vi "Save Last Sync to File.vi"(8 "error in (no error)":errorcluster, 11 "Data Manager in":refnum<class "Data Manager.lvclass">) -> (0 "error out":errorcluster, 3 "Data Manager out":refnum<class "Data Manager.lvclass">)   [LabVIEW 2020, in "Data Manager.lvclass"]
uses:
  Data Manager.lvclass
  Data Manager.lvclass/Data Manager.ctl
  <vilib>/drjdpowell/SQLite Library/SQL Connection/Execute SQL (No results).vi
  <vilib>/drjdpowell/SQLite Library/SQLite.lvlib
  <vilib>/drjdpowell/SQLite Library/SQL Connection/Connection.lvclass
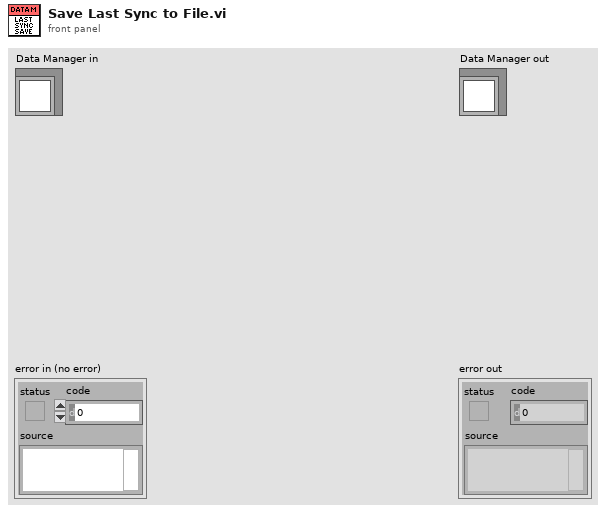
[diagram p1: front panel]
types:
  T1 = typedef "Data Manager.lvclass/Strava JSON for Club Activities--cluster.ctl" = cluster{"athlete":cluster{"firstname":string, "lastname":string}, "type":string, "distance":dbl, "moving_time":dbl, "elapsed_time":dbl, "total_elevation_gain":dbl}
  T2 = typedef "Data Manager.lvclass/Name--cluster.ctl" = cluster{"First":string, "Last":string}
  T3 = typedef "Data Manager.lvclass/Profile--cluster.ctl" = cluster{"Alias":string, "Team":string}
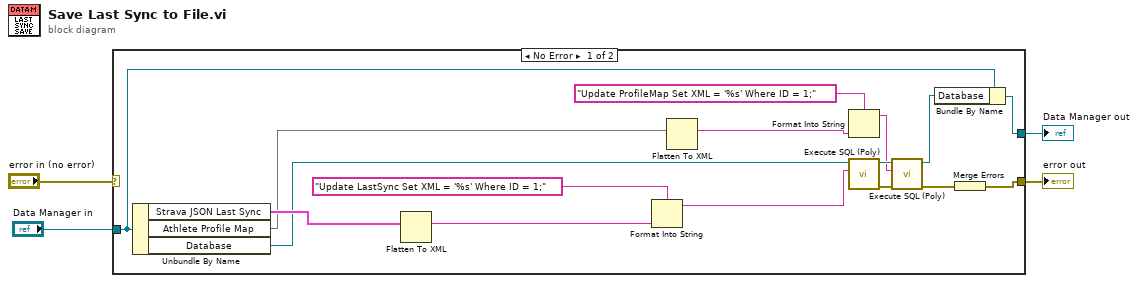
[diagram p0: block diagram]
diagram:
  n1 = case shown="No Error" "error in (no error)" {
    selector: "error in (no error)" -> [_ w22]
    tunnel: [w20 w22] -> w3
    tunnel: [w7 w21] -> w1
    tunnel: "Data Manager in" -> [w8 w21]
    frame No Error {
      n2 = Unbundle By Name(w8) -> ("Strava JSON Last Sync"=w19:T1, "Athlete Profile Map"=w13:map{T2, T3}, "Database"=w9:refnum<class "Connection.lvclass">)
      n3 = Flatten To XML(6:w19) -> (2:w17:string)
      n4 = Format Into String(format string="Update LastSync Set XML = '%s' Where ID = 1;", w17) -> (resulting string=w16:string)  [unwired: 2 in, 1 out]
      n5 = Flatten To XML(6:w13) -> (2:w12:string)
      n6 = Format Into String(format string="Update ProfileMap Set XML = '%s' Where ID = 1;", w12) -> (resulting string=w11:string)  [unwired: 2 in, 1 out]
      n7 = call-poly <vilib>:"Execute SQL (Poly).vi"("SQL"=w16, "SQLite Connection in"=w9) -> ("error out"=w10:errorcluster, "SQLite Connection"=w15:refnum<class "Connection.lvclass">)  [unwired: 8 in]
      n8 = call-poly <vilib>:"Execute SQL (Poly).vi"("error in (no error)"=w10, "SQL"=w11, "SQLite Connection in"=w15) -> ("error out"=w5:errorcluster, "SQLite Connection"=w6:refnum<class "Connection.lvclass">)  [unwired: 7 in]
      n9 = Bundle By Name(cluster=w8, "Database"=w6) -> (w7:refnum<class "Data Manager.lvclass">)
      n10 = Merge Errors(w5) -> (w20:errorcluster)
    }
    frame Error {
    }
  }
  "error out" <- w3
  "Data Manager out" <- w1
